vi "ChannelSettingsQuery.vi"(8 "error in":errorcluster, 11 "T560Object in":refnum<class "T560Channel.lvclass">) -> (0 "error out":errorcluster, 3 "T560Object out":refnum<class "T560Channel.lvclass">)   [LabVIEW 2020, in "T560Channel.lvclass"]
uses:
  T560Channel.lvclass
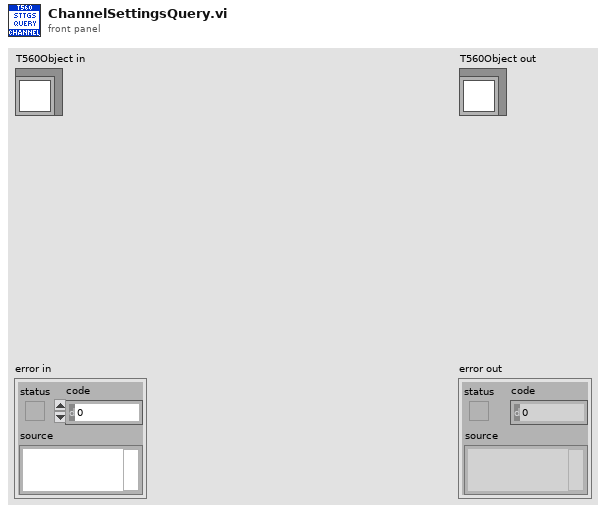
[diagram p1: front panel]
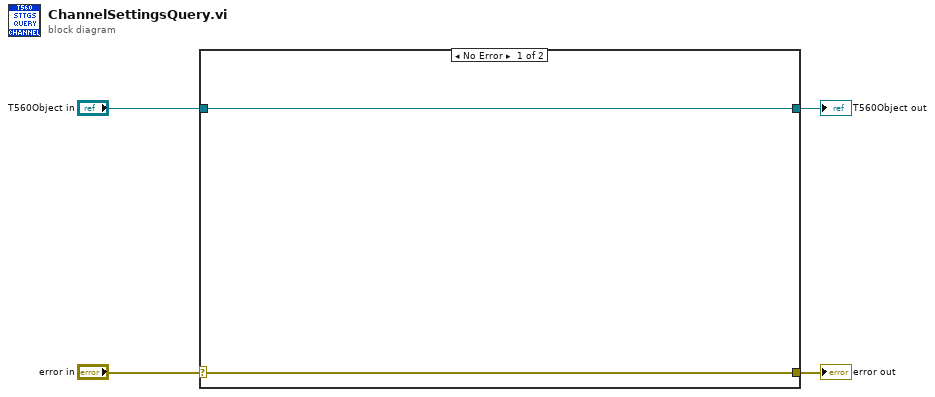
[diagram p0: block diagram]
diagram:
  n1 = case shown="No Error" "error in" {
    selector: "error in" -> [w5 w8]
    tunnel: [w5 w8] -> w3
    tunnel: [w6 w7] -> w1
    tunnel: "T560Object in" -> [w6 w7]
    frame No Error {
    }
    frame Error {
    }
  }
  "error out" <- w3
  "T560Object out" <- w1
